vi "Write U8 FIFO.vi"(6 "FIFO Timestamps":T1, 8 "error in (no error)":errorcluster, 9 "Timeout (ms)":i32, 10 "Data in":u8[](array[numeric]), 11 "CIFFIFO in":refnum<class "CIF_CIPC_Fifo_U8.lvclass">) -> (0 "error out":errorcluster, 1 "timed out?":bool, 2 "Data out":u8[](array[numeric]), 3 "CIFFIFO out":refnum<class "CIF_CIPC_Fifo_U8.lvclass">)   [LabVIEW 2021, in "CIF_CIPC_Fifo_U8.lvclass"]
uses:
  CIF_CIPC_Fifo_U8.lvclass
  CIF_CIPC_Fifo_U8.lvclass/CIF_CIPC_Fifo_U8.ctl
  CIFChannels/CIFChannels.lvclass
  D:/dev/Packages/CIF_Channels_Core/src/CIPC_Channels/CIF_CIPC_Chan/CIF_CIPC_Chn.lvclass
  D:/dev/Packages/CIF_Channels_Core/src/CIFChannels/CIFChannels.lvclass
  D:/dev/Packages/CIF_Channels_Core/src/CIPC_Channels/FIFO_U8/CIF_CIPC_Fifo_U8.lvclass
  ChannelCommon/typedef/TimeStamps.ctl
  ChannelCommon/ChannelCommon.lvlib
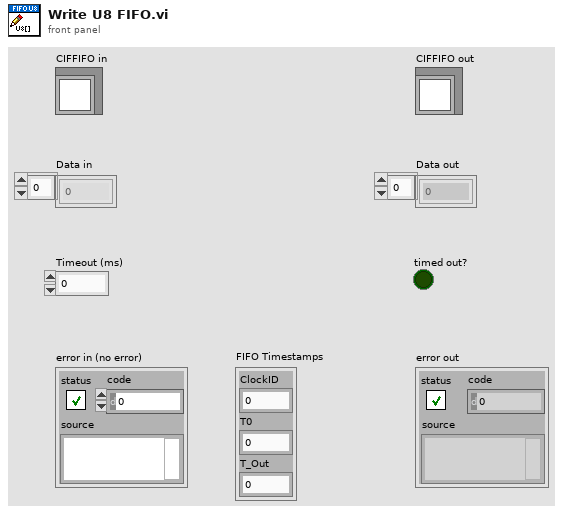
[diagram p1: front panel]
types:
  T1 = typedef "ChannelCommon.lvlib/TimeStamps.ctl" = cluster{"ClockID":u8, "T0":i64, "T_Out":i64}
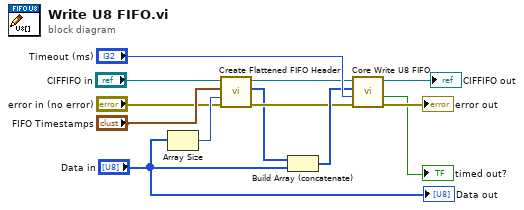
[diagram p0: block diagram]
diagram:
  n1 = Array Size(array="Data in") -> (size(s)=w4:i32)
  n2 = call "Create Flattened FIFO Header.vi"("error in (no error)"="error in (no error)", "Data Length"=w4, "FIFO Timestamps"="FIFO Timestamps", "CIFChannels in"="CIFFIFO in") -> ("error out"=w8:errorcluster, "Flattened FIFO Header"=w6:u8[], "CIFChannels out"=w7:refnum<class "CIF_CIPC_Fifo_U8.lvclass">)  [unwired: 5 in]
  n3 = Build Array (concatenate)(w6, "Data in") -> (w9:u8[])
  n4 = call "Core Write U8 FIFO.vi"("error in (no error)"=w8, "Timeout (ms)"="Timeout (ms)", "U8 With Header in"=w9, "CIFFIFO in"=w7) -> ("error out"=→"error out":errorcluster, "timed out?"=→"timed out?":bool, "CIFFIFO out"=→"CIFFIFO out":refnum<class "CIF_CIPC_Fifo_U8.lvclass">)  [unwired: 4 in, 1 out]
  "Data out" <- "Data in"
